vi "Load waveform and output demo 2.vi"() -> ()   [LabVIEW 2015]
uses:
  <vilib>/Platform/TimedLoop/XDataNode/timing_clust.ctl
  <vilib>/Platform/TimedLoop/XDataNode/nitl_modes.ctl
  <vilib>/Platform/TimedLoop/XDataNode/wakeup.ctl
  <vilib>/rvi/Emulation/niFpgaGetClockAttributes.vi
  <vilib>/rvi/Emulation/niFpgaSctlEmulationGetInTimedLoop.vi
  <vilib>/rvi/Emulation/niFpgaEmulationReportErrorSimple.vi
  <vilib>/rvi/Emulation/niFpgaCriticalErrorInLSC.vi
  <vilib>/rvi/Emulation/niFpgaProcessEmulError.vi
  <vilib>/rvi/DataTransferAndStorage/Container/Common/niFpgaContainerExecOnDevCompGetState.vi
  <vilib>/rvi/DataTransferAndStorage/Container/Common/niFpgaContainerGetUniqueNameForEmu.vi
  <vilib>/rvi/Memory/Memory_Emulation/niFpgaMemoryEmulationDramWriteAndRequestDataApplyByteEnables.vi
  <vilib>/rvi/Memory/Memory_Emulation/niFpgaMemoryEmulationCacheClearOnFirstRun.vi
  <vilib>/rvi/Memory/Memory_Emulation/nirvimemoryEmulationManagerCache_MakeExclusive.vi
  <vilib>/rvi/Memory/Memory_Emulation/nirvimemoryEmulationManagerCache_GetValue.vi
  <vilib>/rvi/Memory/Memory_Emulation/nirvimemoryEmulationManagerCache_InsertValue.vi
  <vilib>/Utility/error.llb/Clear Errors.vi
  <vilib>/rvi/Memory/Memory_Emulation/nirvimemoryEmulationManagerCache_ReleaseExclusive.vi
  <vilib>/rvi/Memory/Memory_Emulation/nirvimemoryEmulationManagerCache_SetValue.vi
  <vilib>/rvi/Emulation/niFpgaEmulationIsFPGAContextNoSignature.vi
  <vilib>/rvi/errors/niFpgaSetErrorForExecOnDevCompSimple.vi
  <vilib>/rvi/eio/common/nirviEmuReportErrorAndStop.vi
  <vilib>/rvi/FIFO/Fifo_Resource/nirvififoEmulationSetSize.vi
  <vilib>/rvi/FIFO/Fifo_Resource/nirviFifoEmulationQueueMgr.vi
  <instcachedir>/0/nirviFifoEmulationQueueMgr_E5CAEC123FF24DC58D834DCA3CDAA9B5.lvgen/nirviFifoEmulationQueueMgr_E5CAEC123FF24DC58D834DCA3CDAA9B5_014.vi
  <vilib>/rvi/FIFO/Fifo_Resource/nirvififoEmulationDetermineInputValidOut.vi
  <vilib>/rvi/FIFO/Fifo_Resource/nirvififoEmulationCreateLock.vi
  <vilib>/rvi/FIFO/Fifo_Resource/nirvififoEmulationObtainLock.vi
  <vilib>/rvi/FIFO/Fifo_Resource/nirvififoEmulationReleaseLock.vi
  <vilib>/rvi/occurrence/nirviWaitOnOccurrenceBase.vi
  <vilib>/rvi/errors/nirviReportUnexpectedCaseInternalError.vi
  <vilib>/rvi/errors/nirviReportUnexpectedCaseInternalError (U32).vi
  <vilib>/rvi/interface/RandomDataEmulation/niFpgaRandomDataHandleErrors.vi
  <vilib>/Platform/TimedLoop/XDataNode/XDataNode.xnode
  <vilib>/rvi/DataTransferAndStorage/Container/XNode/niFpgaContainer.xnode
  <vilib>/rvi/Memory/Memory_Emulation/niFpgaMemoryEmulationDramWriteAndRequestDataRefIn.vi
  <vilib>/rvi/Memory/Memory_Emulation/niFpgaMemoryEmulationDramRetrieveDataRefIn.vi
  <vilib>/rvi/FIFO/Fifo_Resource/niFpgaFifoEmulationRefIn.vi
  <vilib>/Platform/TimedLoop/XDataNode/XDNodeRunTimeDep.lvlib
panel:
  out "Request Done":bool
  out "First E R":u16[](array[numeric])
  in  "Current index":i32
  out "Read Done":bool
  out "Max request address":u32
  out "Last E R":u16[](array[numeric])
  out "First E W":u16[](array[numeric])
  out "Write Done":bool
  out "Max wave DRAM address":u32
  out "Last element written":u16[](array[numeric])
  in  "U16*32":u16[](array[numeric])=[0, 0, 0, 0, 0, 0, 0, 0, 0, 0, 0, 0, 0, 0, 0, 0, 0, 0, 0, 0, 0, 0, 0, 0, 0, 0, 0, 0, 0, 0, 0, 0]
  in  "Current Process":enum16{"Wait", "Write", "Read", "Stop"}(ring)
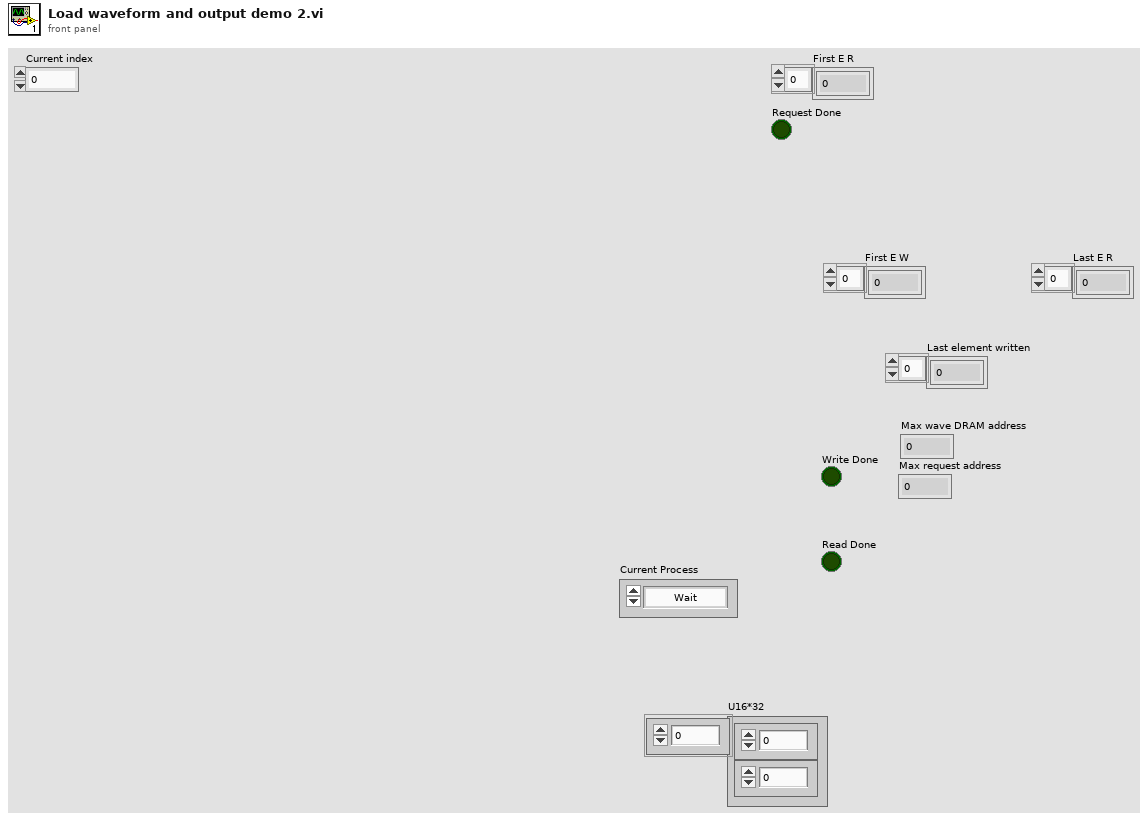
[diagram p1: front panel]
types:
  T1 = typedef "XDNodeRunTimeDep.lvlib/timing_clust.ctl" = cluster{"Expected End [f-1]":u64, "Actual End [f-1]":u64, "Finished Late? [f-1]":bool, "Expected End [i-1]":u64, "Actual End [i-1]":u64, "Finished Late? [i-1]":bool, "Expected Start [i]":u64, "Actual Start [i]":u64, "Expected Start [f]":u64, "Actual Start [f]":u64, "Source Name":string, "Structure Name":string, "Period":i64, "Deadline":i64, "Offset":i64, "Start":i64, "Priority":i32, "Timeout":i32, "Mode":T2, "Wakeup Reason":T3, "Error":errorcluster, "Source Type":string, "Secondary Source Type":string, "Global End Time":u64, "Global Start Time":u64, "Frame Duration":u64, "Iteration Duration":u64, "Assigned CPU":i32, "I/O Scan Engine Mode":u32}
  T2 = typedef "XDNodeRunTimeDep.lvlib/nitl_modes.ctl" = enum32{"No Change", "Process missed periods, maintain original phase", "Discard missed periods, maintain original phase", "Process missed periods, ignore original phase", "Discard missed periods, ignore original phase"}
  T3 = typedef "XDNodeRunTimeDep.lvlib/wakeup.ctl" = enum32{"Normal", "Aborted", "Asynchronous wakeup", "Timing source error", "Timed loop error", "Timeout"}
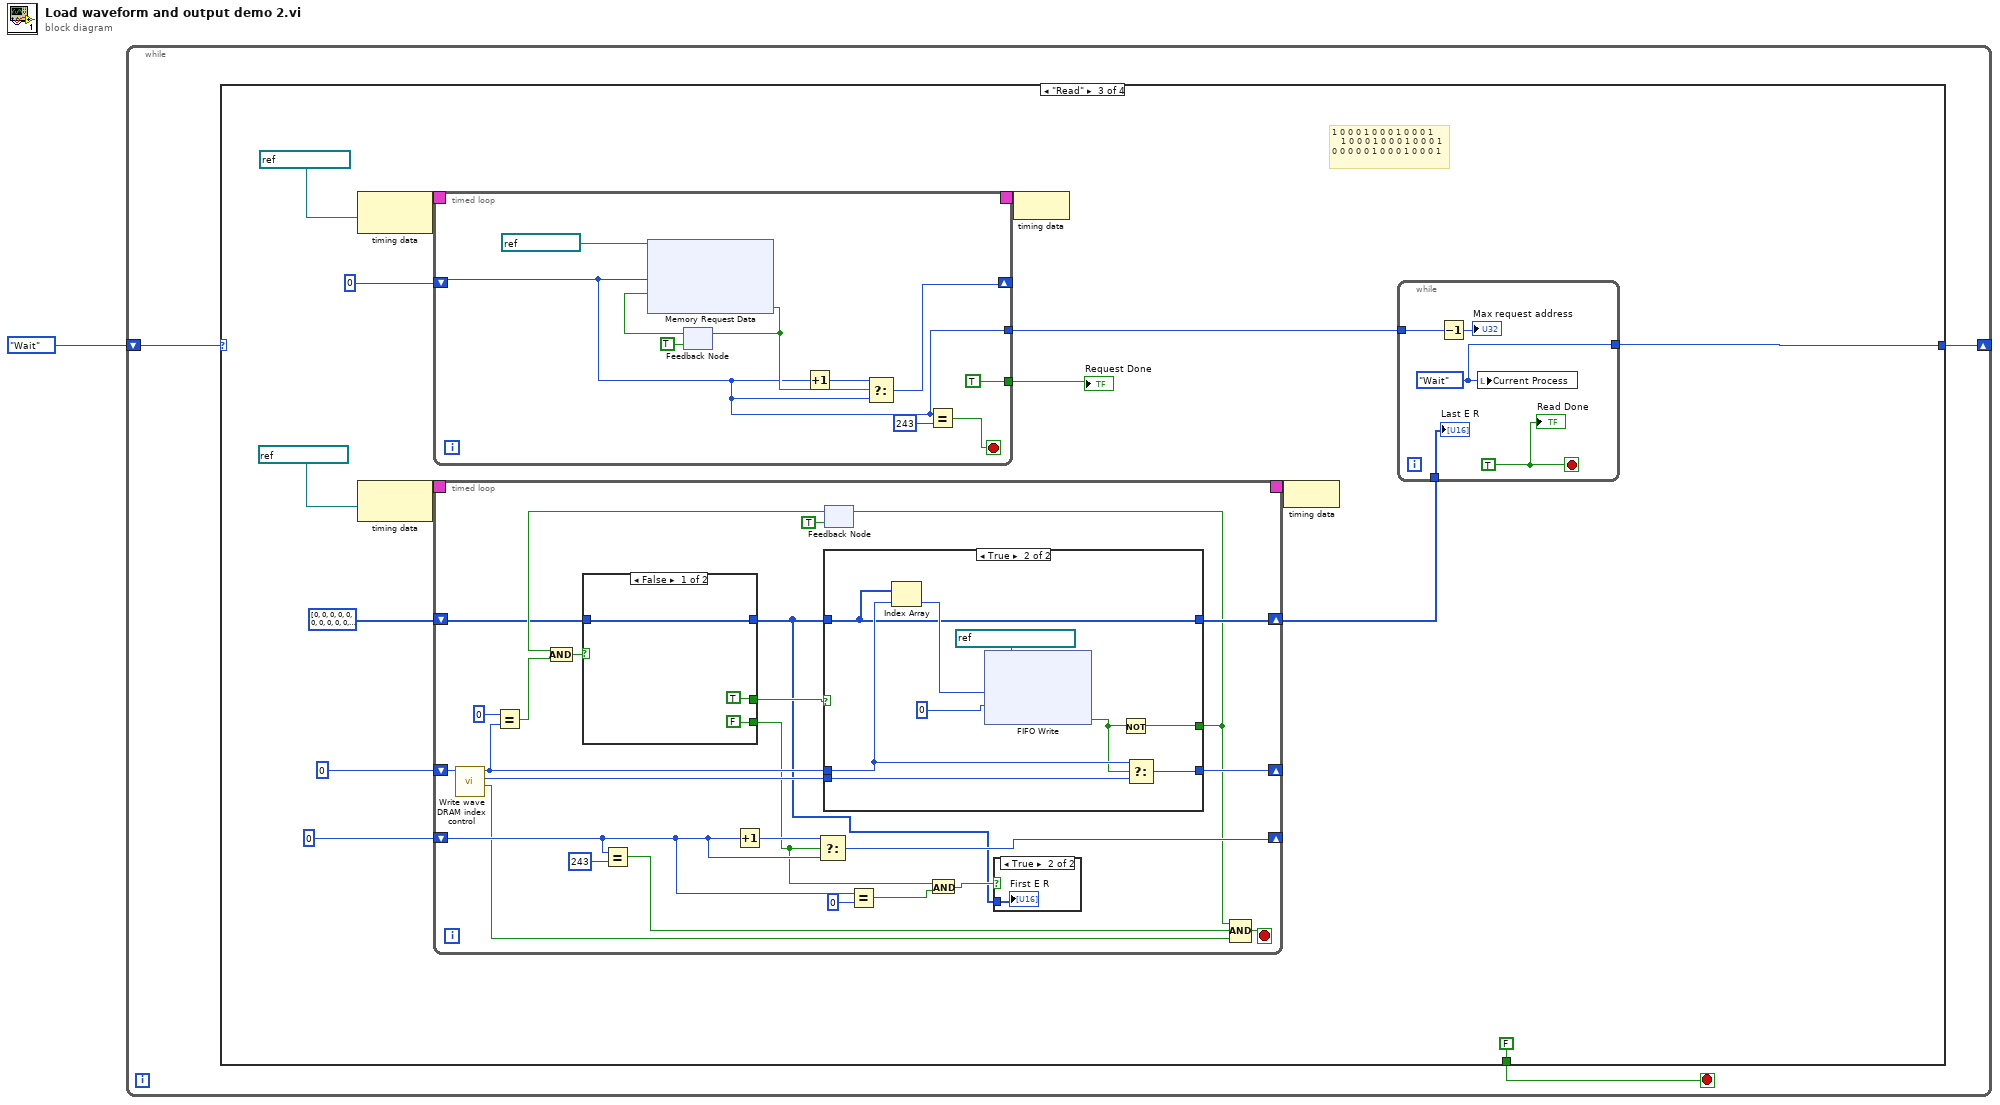
[diagram p0: block diagram]
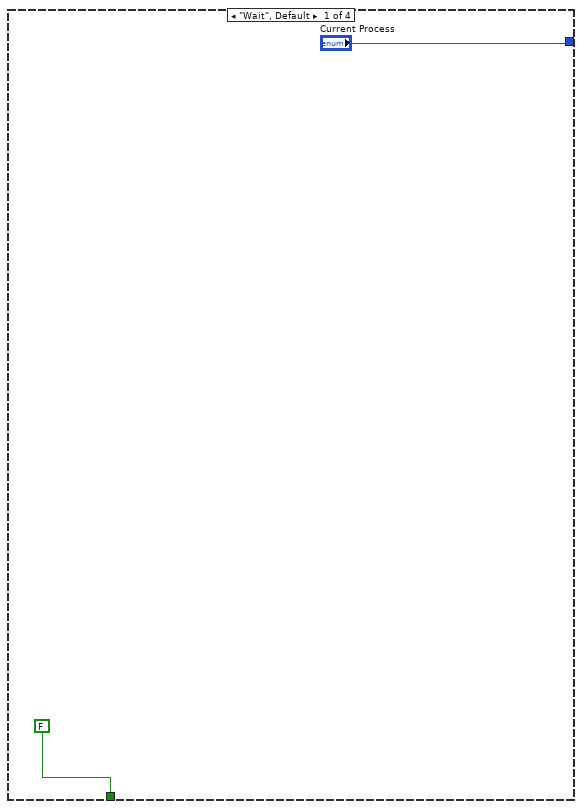
[diagram p2: hidden frame]
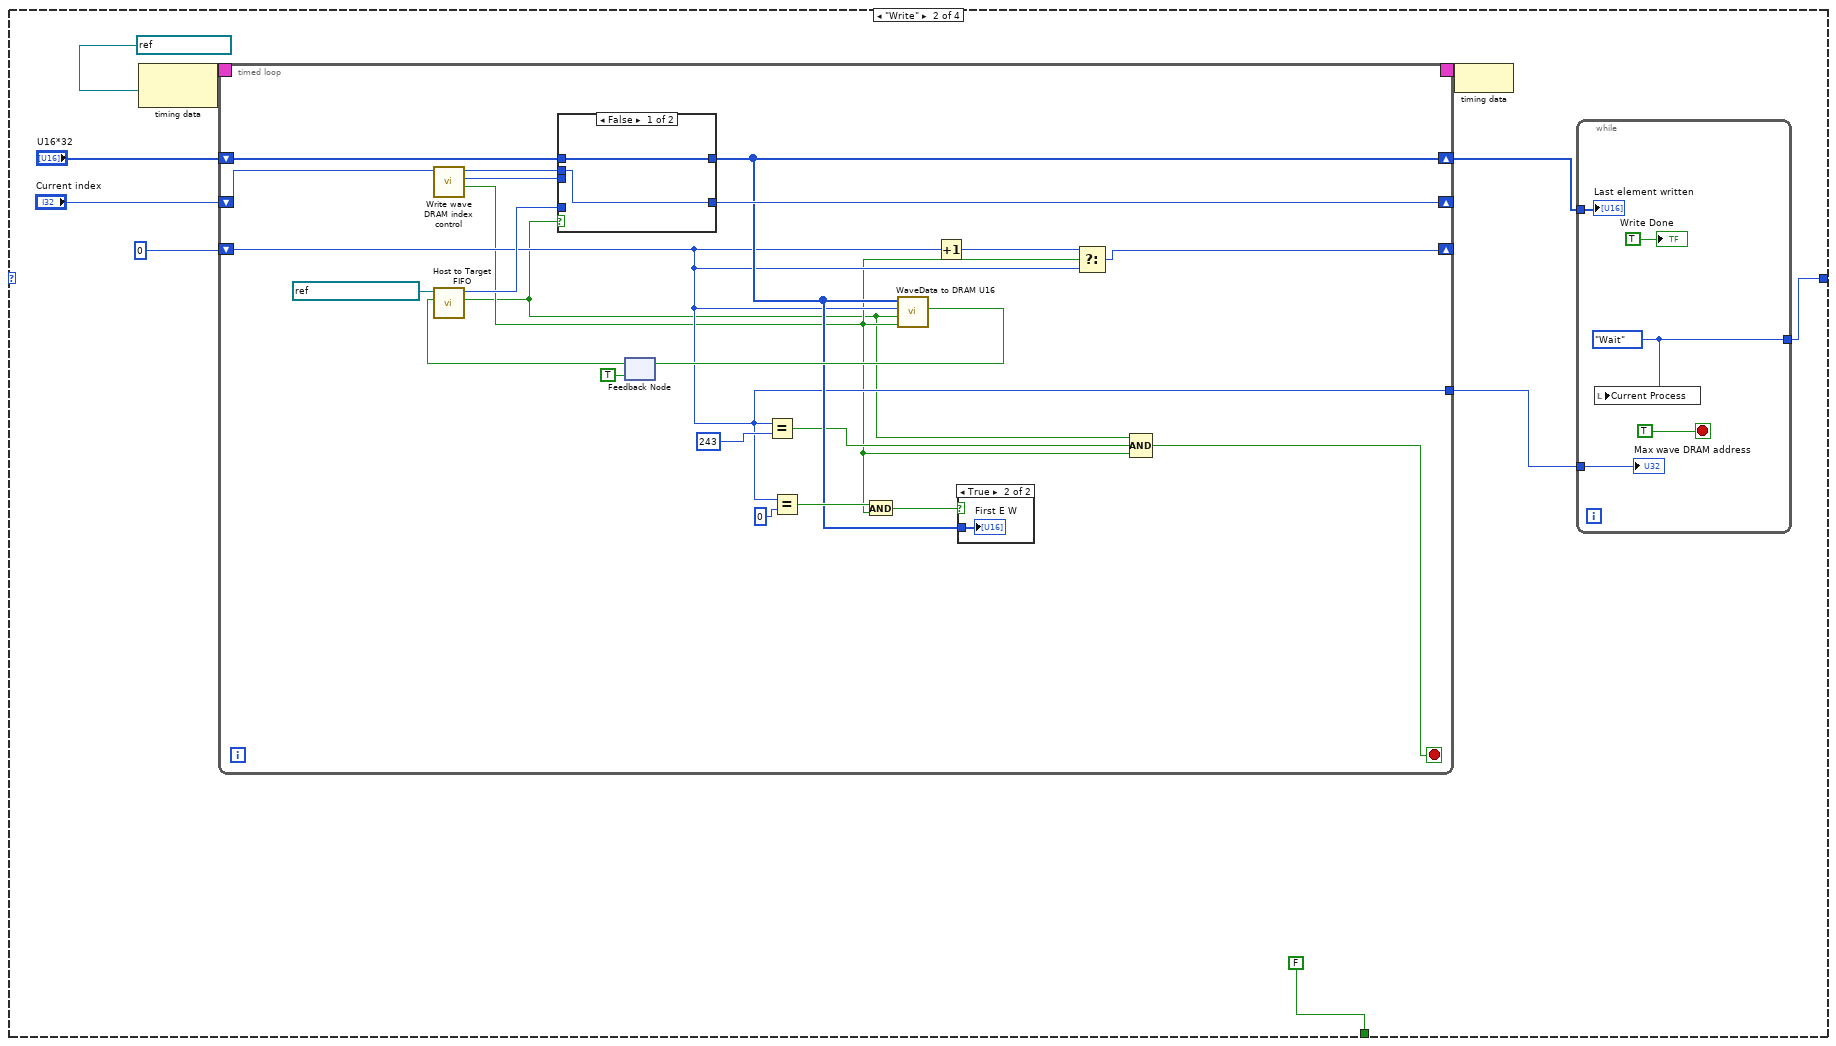
[diagram p3: hidden frame]
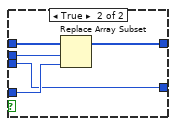
[diagram p5: hidden frame]
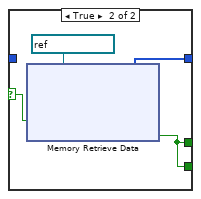
[diagram p7: hidden frame]
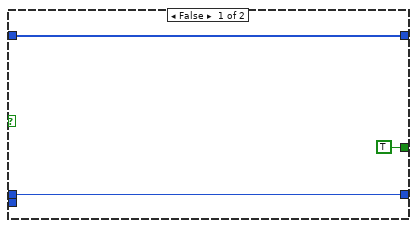
[diagram p8: hidden frame]
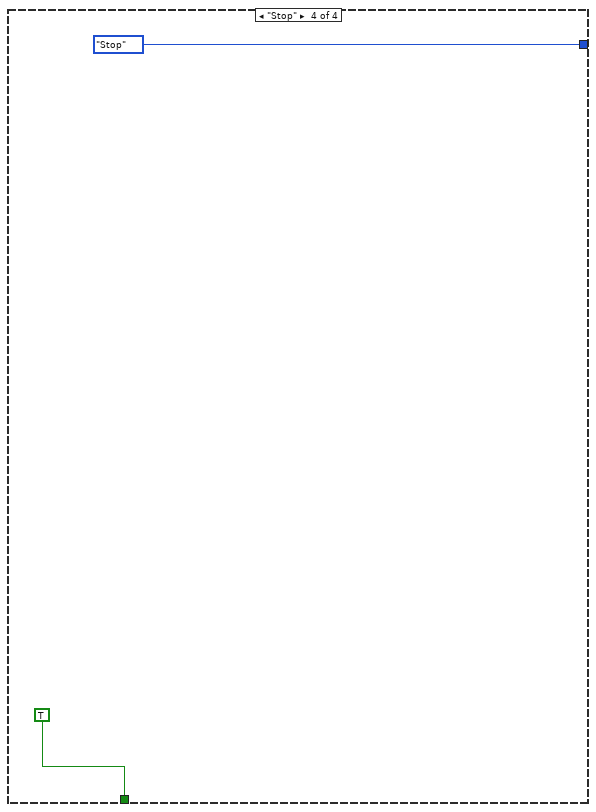
[diagram p9: hidden frame]
diagram:
  n1 = while {
    shift-right: [w4] -> _
    shift-left: enum16{"Wait", "Write", "Read", "Stop"}."Wait" -> [w3]
    stop <- w2 stop-if-true
    n2 = case shown="\"Read\"" w3 {
      tunnel: ["Current Process" w7 w72 enum16{"Wait", "Write", "Read", "Stop"}."Stop" ("Current Process")] -> w4
      tunnel: [FALSE FALSE FALSE TRUE] -> w2
      frame "Wait", Default {
      }
      frame "Write" {
        n3 = node-c288(refnum<k21> "DRAM Clock" ("源名称")) -> (w15:T1)
        n4 = timed-loop {
          timing: w15 -> [_]
          timing-out: [_] -> w14
          shift-right: [w27] -> w9
          shift-left: "U16*32" -> [w42]
          shift-right: [w37] -> _
          shift-left: "Current index" -> [w39]
          shift-right: [w32] -> _
          shift-left: u32 0 ("Address input") -> [w26]
          tunnel: [w26] -> w8
          stop <- w23 stop-if-true
          n5 = call "Write wave DRAM index control.vi"("Current index"=w39) -> ("Output Valid"=w24:bool, "Next index"=w38:i32, "Current index"=w40:i32)  [unwired: 8 in]
          n6 = feedback #1(TRUE ("输入就绪")) -> (w36:bool)
          n7 = call "Host to Target FIFO.vi"("Ready for Input"=w36, "FIFO Name"=refnum<k21> "Host to Target U16") -> ("Output Valid"=w22:bool, "Data"=w41:u16)  [unwired: 8 in]
          n8 = case shown="False" w22 {
            tunnel: w42 -> [w46 w51]
            tunnel: w41 -> [_ w50]
            tunnel: w40 -> [w45 w49]
            tunnel: [w46 w48] -> w27
            tunnel: w38 -> [_ w47]
            tunnel: [w45 w47] -> w37
            frame False {
            }
            frame True {
              n9 = Replace Array Subset(array=w51, new element=w50, index=w49) -> (w48:u16[])
            }
          }
          n10 = Equal?(x=w26, y=u32 243) -> (x = y?=w25:bool)
          n11 = Equal?(x=w26, y=u32 0) -> (x = y?=w29:bool)
          n12 = And(x=w29, y=w24) -> (x .and. y?=w28:bool)
          n13 = call "WaveData to DRAM U16.vi"("input valid? 2"=w24, "input valid?"=w22, "Address input"=w26, "Data"=w27) -> ("Input ready"=w34:bool)  [unwired: 7 in]
          n14 = feedback-in #1(w34) -> ()
          n15 = Increment(x=w26) -> (x+1=w33:u32)
          n16 = case shown="True" w28 {
            tunnel: w27 -> [_ w44]
            frame False {
            }
            frame True {
              "First E W" <- w44
            }
          }
          n17 = Select(t=w33, s=w24, f=w26) -> (s? t:f=w32:u32)
          n18 = Compound Arithmetic op=AND(w22, w25, w24) -> (w23:bool)
        }
        n19 = node-c288(w14) -> ()
        n20 = while {
          tunnel: [w21] -> w7
          tunnel: w9 -> [w18]
          tunnel: w8 -> [w17]
          stop <- TRUE stop-if-true
          w21 = enum16{"Wait", "Write", "Read", "Stop"}."Wait"
          n21 = local write "Current Process"(w21) -> ()
          "Write Done" <- TRUE ("Write Done")
          "Max wave DRAM address" <- w17
          "Last element written" <- w18
        }
      }
      frame "Read" {
        # "1 0 0 0 1 0 0 0 1 0 0 0 1\n   1 0 0 0 1 0 0 0 1 0 0 0 1\n0 0 0 0 0 1 0 0 0 1 0 0 0 1"
        n22 = node-c288(refnum<k21> "DRAM Clock" ("源名称")) -> (w70:T1)
        n23 = node-c288(refnum<k21> "DRAM Clock" ("源名称")) -> (w66:T1)
        n24 = timed-loop {
          timing: w70 -> [_]
          timing-out: [_] -> w69
          shift-right: [w128] -> _
          shift-left: u32 0 ("地址") -> [w125]
          tunnel: [w125] -> w59
          tunnel: [TRUE] -> w58
          stop <- w126 stop-if-true
          n25 = feedback #2(TRUE ("输入就绪")) -> (w130:bool)
          n26 = xnode ("Memory Request Data")("Address"=w125, "Input Valid"=w130, "Memory In"=refnum<k21> "Waveform" ("存储器输入")) -> ("Ready for Input"=w131:bool)  [unwired: 1 out]
          n27 = feedback-in #2(w131) -> ()
          n28 = Increment(x=w125) -> (x+1=w132:u32)
          n29 = Select(t=w132, s=w131, f=w125) -> (s? t:f=w128:u32)
          n30 = Equal?(x=w125, y=u32 243) -> (x = y?=w126:bool)
        }
        "Request Done" <- w58
        n31 = timed-loop {
          timing: w66 -> [_]
          timing-out: [_] -> w65
          shift-right: [w96] -> _
          shift-left: 0 ("Current index") -> [w82]
          shift-right: [w94] -> _
          shift-left: 0 ("Current index") -> [w95]
          shift-right: [w85] -> w60
          shift-left: u16[] [0, 0, 0, 0, 0, 0, 0, 0, 0, 0, 0, 0, 0, 0, 0, 0, 0, 0, 0, 0, 0, 0, 0, 0, 0, 0, 0, 0, 0, 0, 0, 0] ("数据") -> [w84]
          stop <- w75 stop-if-true
          n32 = call "Write wave DRAM index control.vi"("Current index"=w95) -> ("Output Valid"=w73:bool, "Next index"=w93:i32, "Current index"=w91:i32)  [unwired: 8 in]
          n33 = Equal?(x=0, y=w91) -> (x = y?=w87:bool)
          n34 = Equal?(x=w82, y=243) -> (x = y?=w74:bool)
          n35 = Increment(x=w82) -> (x+1=w97:i32)
          n36 = feedback #3(TRUE) -> (w88:bool)
          n37 = And(x=w88, y=w87) -> (x .and. y?=w86:bool)
          n38 = case shown="False" w86 {
            selector: w86 -> [_ w102]
            tunnel: [w99 w104] -> w77
            tunnel: [TRUE w103] -> w92
            tunnel: [FALSE ("输出有效") w103] -> w79
            tunnel: w84 -> [w99 _]
            frame False {
            }
            frame True {
              n39 = xnode ("Memory Retrieve Data")("Ready for Output"=w102, "Memory In"=refnum<k21> "Waveform" ("存储器输入")) -> ("Data"=w104:u16[], "Output Valid"=w103:bool)  [unwired: 1 out]
            }
          }
          n40 = Select(t=w97, s=w79, f=w82) -> (s? t:f=w96:i32)
          n41 = case shown="True" w92 {
            tunnel: w77 -> [w107 w109]
            tunnel: [w108 w114] -> w94
            tunnel: w91 -> [w108 w113]
            tunnel: w93 -> [_ w112]
            tunnel: [TRUE w110] -> w76
            tunnel: [w107 w109] -> w85
            frame False {
            }
            frame True {
              n42 = Index Array(array=w109, index=w113) -> (element=w117:u16)
              n43 = xnode ("FIFO Write")("Element"=w117, "Timeout"=0 ("超时"), "FIFO In"=refnum<k21> "Target to Host U16" ("FIFO输入")) -> ("Timed Out?"=w111:bool)  [unwired: 1 out]
              n44 = Not(x=w111) -> (.not. x?=w110:bool)
              n45 = Select(t=w113, s=w111, f=w112) -> (s? t:f=w114:i32)
            }
          }
          n46 = feedback-in #3(w76) -> ()
          n47 = Equal?(x=w82, y=0) -> (x = y?=w80:bool)
          n48 = And(x=w79, y=w80) -> (x .and. y?=w78:bool)
          n49 = case shown="True" w78 {
            tunnel: w77 -> [_ w98]
            frame False {
            }
            frame True {
              "First E R" <- w98
            }
          }
          n50 = Compound Arithmetic op=AND(w76, w74, w73) -> (w75:bool)
        }
        n51 = node-c288(w69) -> ()
        n52 = node-c288(w65) -> ()
        n53 = while {
          tunnel: [w143] -> w72
          tunnel: w60 -> [w142]
          tunnel: w59 -> [w140]
          stop <- w144 stop-if-true
          w143 = enum16{"Wait", "Write", "Read", "Stop"}."Wait" ("Current Process")
          w144 = TRUE
          n54 = Decrement(x=w140) -> (x-1=→"Max request address":u32)
          n55 = local write "Current Process"(w143) -> ()
          "Read Done" <- w144
          "Last E R" <- w142
        }
      }
      frame "Stop" {
      }
    }
  }
